vi "zeroPadArrayarbitraryLength.vi"(1 "# Zeros":i32, 2 "Array to Pad":dbl[](array[numeric]) format="%.2f") -> (0 "Output Array":dbl[](array[numeric]) format="%.2f")   [LabVIEW 2013]
panel:
  # "Zero Padder\n(Arbitrary Length)"
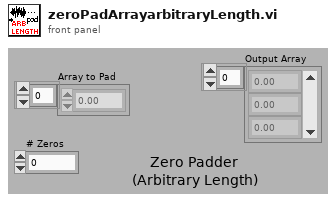
[diagram p1: front panel]
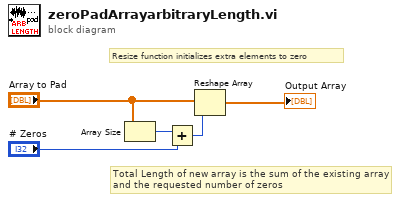
[diagram p0: block diagram]
diagram:
  # "Resize function initializes extra elements to zero"
  # "Total Length of new array is the sum of the existing array\nand the requested number of zeros"
  n1 = Array Size(array="Array to Pad") -> (size(s)=w5:i32)
  n2 = Add(x=w5, y="# Zeros") -> (x+y=w4:i32)
  n3 = Reshape Array("Array to Pad", w4) -> (→"Output Array":dbl[])
